vi "setup Write Motor LV.vi"(9 "value":u16, 10 "motorNum":u8, 11 "instance":i32) -> ()   [LabVIEW 2023, in "SADI_FW3.lvlib"]
doc: "SADI_API_Wrapper void setupWrite_Motor_LV( int instance ,\n uint8_t motorNum ,\n uint16_t value );"
uses:
  SADI_FW3.lvlib
  SADI_FW3.dll
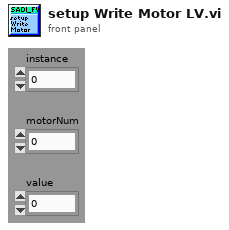
[diagram p1: front panel]
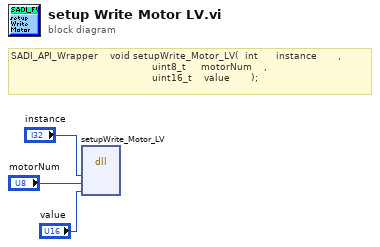
[diagram p0: block diagram]
diagram:
  # "SADI_API_Wrapper    void setupWrite_Motor_LV(  int      instance       ,\n                                               uint8_t     motorNum    ,\n                                               uint16_t    value       );"
  n1 = dll-call lib="C:/Users/loran/Documents/School/24_Spring/Controls Lab/EML4314c_Sp24_framework_0/LVLib/SADI_FW3.*" fn="setupWrite_Motor_LV"("instance"="instance", "motorNum"="motorNum", "value"="value") -> ()  [unwired: 7 in, 2 out]
